vi "Initialize Hardware References.vi"(8 "error in (no error)":errorcluster, 11 "Hardware Resources in":T1={"AI"={"DAQmx Channel"="", "Max Input"=0.0, "Min Input"=0.0, "Sample Rate"=0.0, "DAQmx Task"="", "shunt resistor location"=-1, "external shunt resistor value"=249.0}, "AO"={"DAQmx Channel"="", "Max Output"=0.0, "Min Output"=0.0, "Sample Rate"=0.0, "DAQmx Task"=""}, "DO"={"DAQmx Channel"="", "Sample Rate"=0.0, "DAQmx Task"=""}, "DI"={"DAQmx Channel"="", "Sample Rate"=0.0, "DAQmx Task"=""}, "TC"={"DAQmx Channel"="", "Max Inout"=0.0, "Min Input"=0.0, "Sample Rate"=0.0, "DAQmx Task"="", "resistance configuration"=4, "r0"=100.0, "current excitation value"=0.0025, "current excitation source"=10167, "rtd type"=12481}} {"TC"."rtd type" items=["Pt3750"=12481, "Pt3851"=10071, "Pt3911"=12482, "Pt3916"=10069, "Pt3920"=10053, "Pt3928"=12483, "Custom"=10137]; "TC"."current excitation source" items=["Internal"=10200, "External"=10167, "None"=10230]; "TC"."resistance configuration" items=["2-Wire"=2, "3-Wire"=3, "4-Wire"=4]; "AI"."shunt resistor location" items=["default"=-1, "RSE"=10083, "NRSE"=10078, "Differential"=10106, "Pseudodifferential"=12529]}) -> (0 "error out":errorcluster, 3 "Hardware Resources out":T1={"AI"={"DAQmx Channel"="", "Max Input"=0.0, "Min Input"=0.0, "Sample Rate"=0.0, "DAQmx Task"="", "shunt resistor location"=-1, "external shunt resistor value"=249.0}, "AO"={"DAQmx Channel"="", "Max Output"=0.0, "Min Output"=0.0, "Sample Rate"=0.0, "DAQmx Task"=""}, "DO"={"DAQmx Channel"="", "Sample Rate"=0.0, "DAQmx Task"=""}, "DI"={"DAQmx Channel"="", "Sample Rate"=0.0, "DAQmx Task"=""}, "TC"={"DAQmx Channel"="", "Max Inout"=0.0, "Min Input"=0.0, "Sample Rate"=0.0, "DAQmx Task"="", "resistance configuration"=4, "r0"=100.0, "current excitation value"=0.0025, "current excitation source"=10167, "rtd type"=12481}} {"TC"."rtd type" items=["Pt3750"=12481, "Pt3851"=10071, "Pt3911"=12482, "Pt3916"=10069, "Pt3920"=10053, "Pt3928"=12483, "Custom"=10137]; "TC"."current excitation source" items=["Internal"=10200, "External"=10167, "None"=10230]; "TC"."resistance configuration" items=["2-Wire"=2, "3-Wire"=3, "4-Wire"=4]; "AI"."shunt resistor location" items=["default"=-1, "RSE"=10083, "NRSE"=10078, "Differential"=10106, "Pseudodifferential"=12529]})   [LabVIEW 2024, in "Acquisition.lvlib"]
doc: "Initialize the hardware references."
uses:
  Acquisition.lvlib
  Hardware Configuration.ctl
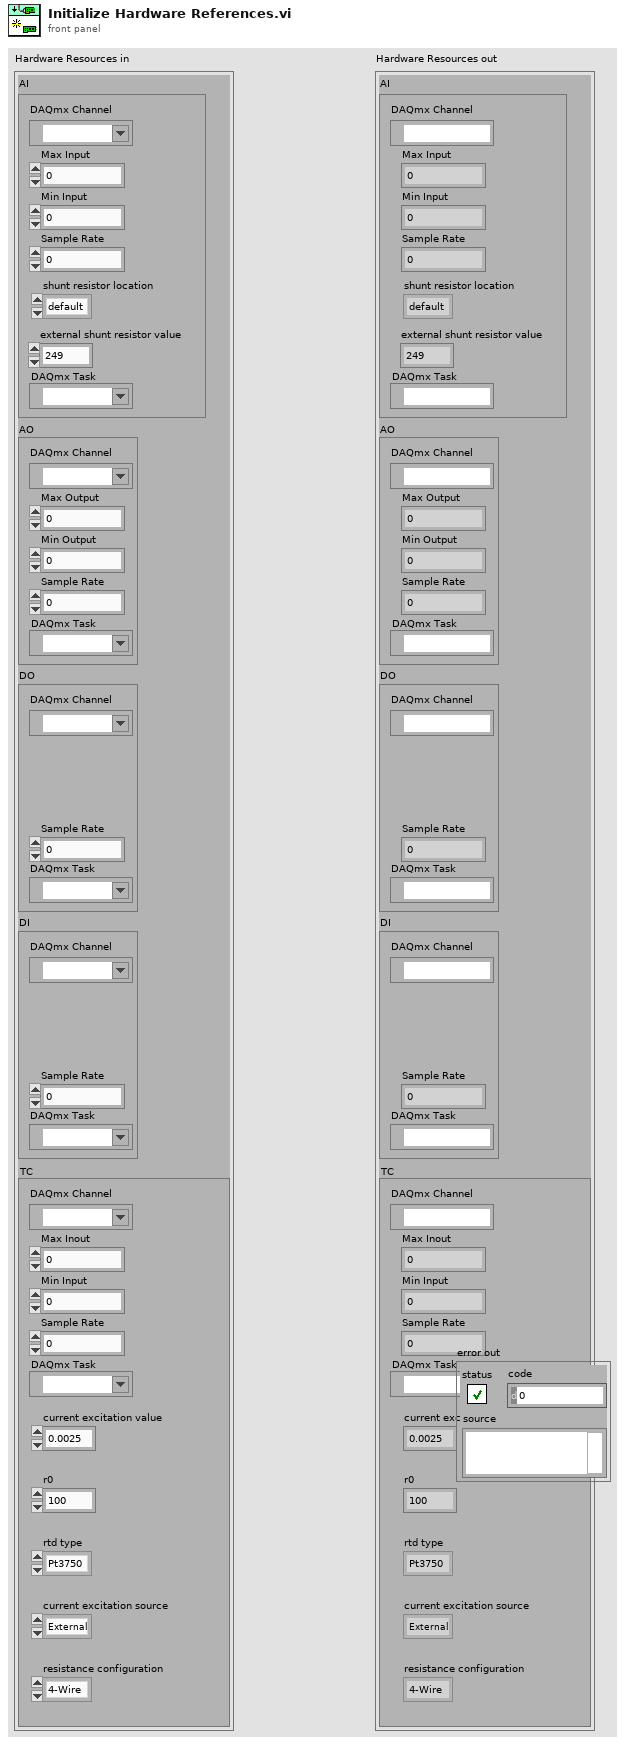
[diagram p1: front panel]
types:
  T1 = typedef "Acquisition.lvlib/Hardware Configuration.ctl" = cluster{"AI":cluster{"DAQmx Channel":tag, "Max Input":dbl, "Min Input":dbl, "Sample Rate":dbl, "DAQmx Task":refnum<k21>, "shunt resistor location":i32, "external shunt resistor value":dbl}, "AO":cluster{"DAQmx Channel":tag, "Max Output":dbl, "Min Output":dbl, "Sample Rate":dbl, "DAQmx Task":refnum<k21>}, "DO":cluster{"DAQmx Channel":tag, "Sample Rate":dbl, "DAQmx Task":refnum<k21>}, "DI":cluster{"DAQmx Channel":tag, "Sample Rate":dbl, "DAQmx Task":refnum<k21>}, "TC":cluster{"DAQmx Channel":tag, "Max Inout":dbl, "Min Input":dbl, "Sample Rate":dbl, "DAQmx Task":refnum<k21>, "resistance configuration":i32, "r0":dbl, "current excitation value":dbl, "current excitation source":i32, "rtd type":i32}}
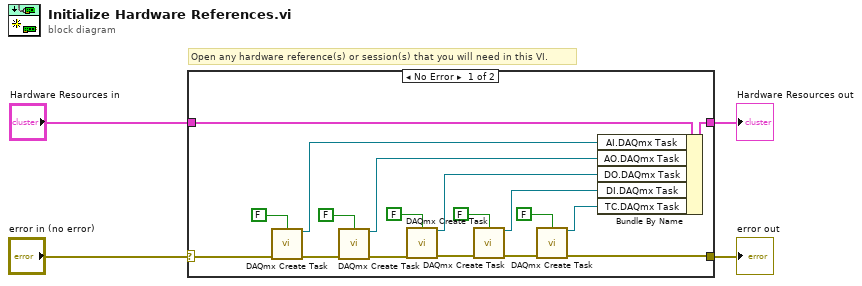
[diagram p0: block diagram]
diagram:
  # "Open any hardware reference(s) or session(s) that you will need in this VI."
  n1 = case shown="No Error" "error in (no error)" {
    selector: "error in (no error)" -> [w15 w23]
    tunnel: [w10 w23] -> w3
    tunnel: "Hardware Resources in" -> [w21 w24]
    tunnel: [w22 w24] -> w1
    frame No Error {
      n2 = call <vilib>:"DAQmx Create Task.vi"("auto cleanup"=FALSE, "error in"=w15) -> ("task out"=w9:refnum<k21>, "error out"=w14:errorcluster)  [unwired: 12 in]
      n3 = call <vilib>:"DAQmx Create Task.vi"("auto cleanup"=FALSE, "error in"=w14) -> ("task out"=w8:refnum<k21>, "error out"=w13:errorcluster)  [unwired: 12 in]
      n4 = call <vilib>:"DAQmx Create Task.vi"("auto cleanup"=FALSE, "error in"=w13) -> ("task out"=w7:refnum<k21>, "error out"=w12:errorcluster)  [unwired: 12 in]
      n5 = call <vilib>:"DAQmx Create Task.vi"("auto cleanup"=FALSE, "error in"=w12) -> ("task out"=w6:refnum<k21>, "error out"=w11:errorcluster)  [unwired: 12 in]
      n6 = call <vilib>:"DAQmx Create Task.vi"("auto cleanup"=FALSE, "error in"=w11) -> ("task out"=w5:refnum<k21>, "error out"=w10:errorcluster)  [unwired: 12 in]
      n7 = Bundle By Name(cluster=w21, "AI.DAQmx Task"=w9, "AO.DAQmx Task"=w8, "DO.DAQmx Task"=w7, "DI.DAQmx Task"=w6, "TC.DAQmx Task"=w5) -> (w22:T1)
    }
    frame Error {
    }
  }
  "Hardware Resources out" <- w1
  "error out" <- w3
